vi "Set FPGA Mode.vi"(8 "error in (no error)":errorcluster, 10 "FPGAScanInterfaceMode":T2, 11 "Item Ref in":T1 format="%.0x") -> (0 "error out":errorcluster, 3 "Item Ref out":T1 format="%.0x")   [LabVIEW 2017, in "Scan Engine Custom Device.lvlib"]
uses:
  Scan Engine Custom Device.lvlib
  Type Defs/Host - FPGAScanInterfaceMode.ctl
  <vilib>/NI Veristand/Custom Device API/Custom Device Item Ref.ctl
  NationalInstruments.VeriStand.SystemDefinitionAPI
  <vilib>/NI Veristand/Custom Device Tools/Custom Device Utility Library/Custom Device Utility Library.lvlib
  <vilib>/NI Veristand/Custom Device Offline API/Custom Device Offline API.lvlib
  <vilib>/NI Veristand/Custom Device API/Custom Device API.lvlib
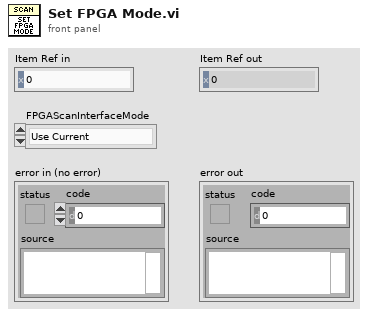
[diagram p1: front panel]
types:
  T1 = typedef "Custom Device API.lvlib/Custom Device Item Ref.ctl" = u64
  T2 = typedef "Scan Engine Custom Device.lvlib/Host - FPGAScanInterfaceMode.ctl" = enum16{"Use Current", "FPGA", "Scan Mode"}
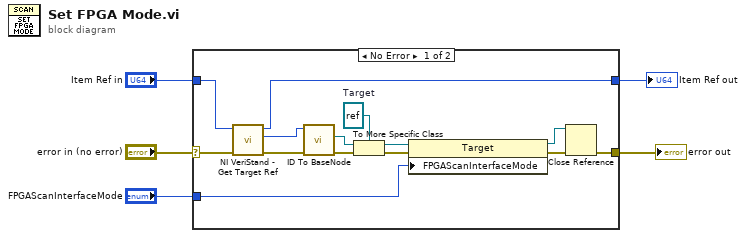
[diagram p0: block diagram]
diagram:
  n1 = case shown="No Error" "error in (no error)" {
    selector: "error in (no error)" -> [w6 w20]
    tunnel: [w19 w20] -> w5
    tunnel: "FPGAScanInterfaceMode" -> [w16 _]
    tunnel: [w10 w21] -> w3
    tunnel: "Item Ref in" -> [w7 w21]
    frame No Error {
      w12 = refnum<k24> refnum  # Target
      n2 = call <vilib>:"NI VeriStand - Get Target Ref.vi"("error in"=w6, "Item Ref in"=w7) -> ("error out"=w8:errorcluster, "Target Ref"=w9:T1, "Item Ref out"=w10:T1)  [unwired: 6 in, 1 out]
      n3 = call <vilib>:"ID To BaseNode.vi"("error in (no error)"=w8, "ID in"=w9) -> ("error out"=w15:errorcluster, "BaseNode"=w11:refnum<k24>)  [unwired: 7 in, 1 out]
      n4 = To More Specific Class(target class=w12, reference=w11, error in=w15) -> (specific class reference=w13:refnum<k24>, error out=w14:errorcluster)
      n5 = property class="Target"(reference=w13, error in=w14, "FPGAScanInterfaceMode"=w16) -> (reference out=w18:refnum<k24>, error out=w17:errorcluster)
      n6 = Close Reference(reference=w18, error in (no error)=w17) -> (error out=w19:errorcluster)
    }
    frame Error {
    }
  }
  "error out" <- w5
  "Item Ref out" <- w3
